vi "Update Configuration Revision.vi"(8 "error in (no error)":errorcluster, 11 "Hardware Ref in":T1 format="%.0x") -> (0 "error out":errorcluster, 3 "Hardware Ref out":T1 format="%.0x")   [LabVIEW 2020, in "Routing and Faulting Hardware API.lvlib"]
uses:
  Routing and Faulting Hardware API.lvlib
  <vilib>/NI VeriStand/Custom Device API/Custom Device Item Ref.ctl
  <vilib>/NI VeriStand/Custom Device API/Custom Device API.lvlib
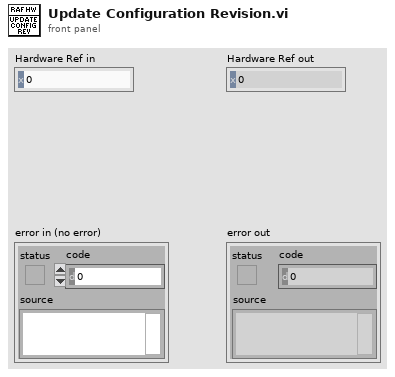
[diagram p1: front panel]
types:
  T1 = typedef "Custom Device API.lvlib/Custom Device Item Ref.ctl" = u64
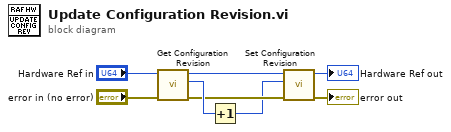
[diagram p0: block diagram]
diagram:
  n1 = call "Get Configuration Revision.vi"("error in (no error)"="error in (no error)", "Hardware Ref in"="Hardware Ref in") -> ("error out"=w5:errorcluster, "Configuration Revision"=w6:u32, "Hardware Ref out"=w3:T1)  [unwired: 6 in, 1 out]
  n2 = Increment(x=w6) -> (x+1=w1:u32)
  n3 = call "Set Configuration Revision.vi"("error in (no error)"=w5, "Configuration Revision"=w1, "Hardware Ref in"=w3) -> ("error out"=→"error out":errorcluster, "Hardware Ref out"=→"Hardware Ref out":T1)  [unwired: 7 in]
